vi "Native POST Multipart File Upload Example.vi"() -> ()   [LabVIEW 2017]
uses:
  <vilib>/httpClient/MultipartData.ctl
  <vilib>/httpClient/LabVIEWHTTPClient.lvlib
panel:
  out "body":string
  out "headers":string
  in  "Authentication":cluster{"Username":string, "Password":string}
  out "error out":errorcluster
  in  "FIlepath":path=path "D:/upwork/Labview-REST-API/labview-source/payload.png"
  in  "API Endpoint Url":string="https://luferau.free.beeceptor.com/upload"
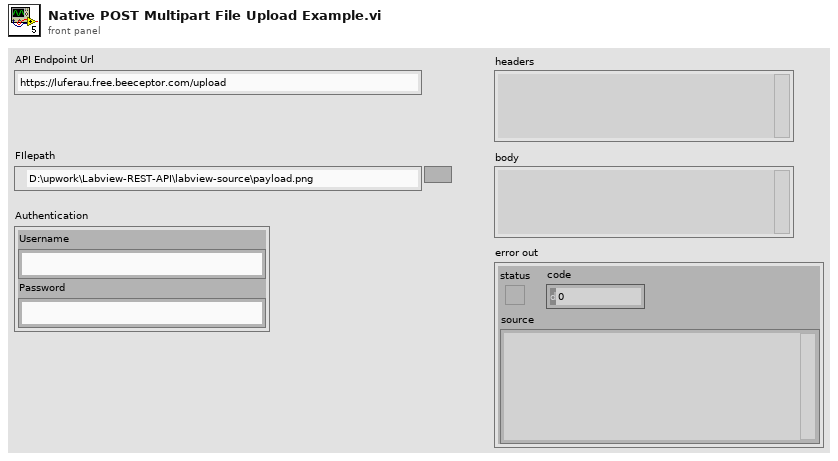
[diagram p1: front panel]
types:
  T1 = typedef "LabVIEWHTTPClient.lvlib/MultipartData.ctl" = cluster{"Name":string, "Value":string, "File":path, "Filename":string, "MIME type":string}
  T2 = typedef "LabVIEWHTTPClient.lvlib/ClientHandle.ctl" = refnum<k1>
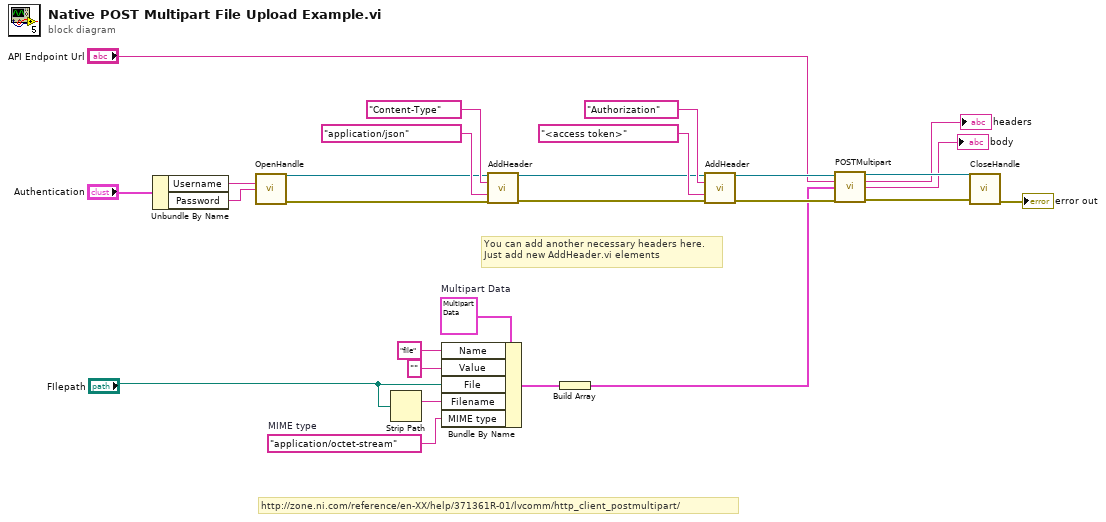
[diagram p0: block diagram]
diagram:
  w4 = "application/octet-stream"  # MIME type
  w8 = T1 {"Name"="", "Value"="", "File"=path "", "Filename"="", "MIME type"="application/octet-stream"}  # Multipart Data
  # "http://zone.ni.com/reference/en-XX/help/371361R-01/lvcomm/http_client_postmultipart/"
  # "You can add another necessary headers here.\nJust add new AddHeader.vi elements"
  n1 = Unbundle By Name("Authentication") -> ("Username"=w26:string, "Password"=w25:string)
  n2 = call <vilib>:"OpenHandle.vi"("username"=w26, "password"=w25) -> ("client handle out"=w10:T2, "error out"=w13:errorcluster)  [unwired: 12 in]
  n3 = Strip Path(path="FIlepath") -> (name=w5:string)  [unwired: 1 out]
  n4 = Bundle By Name(cluster=w8, "Name"="file", "Value"="", "File"="FIlepath", "Filename"=w5, "MIME type"=w4) -> (w3:T1)
  n5 = call <vilib>:"AddHeader.vi"("client handle"=w10, "header"="Content-Type", "value"="application/json", "error in (no error)"=w13) -> ("client handle out"=w11:T2, "error out"=w12:errorcluster)  [unwired: 10 in]
  n6 = Build Array(w3) -> (w1:T1[])
  n7 = call <vilib>:"AddHeader.vi"("client handle"=w11, "header"="Authorization", "value"="<access token>", "error in (no error)"=w12) -> ("client handle out"=w21:T2, "error out"=w20:errorcluster)  [unwired: 10 in]
  n8 = call <vilib>:"POSTMultipart.vi"("client handle"=w21, "url"="API Endpoint Url", "data"=w1, "error in (no error)"=w20) -> ("client handle out"=w19:T2, "headers"=→"headers":string, "body"=→"body":string, "error out"=w18:errorcluster)  [unwired: 8 in]
  n9 = call <vilib>:"CloseHandle.vi"("client handle"=w19, "error in (no error)"=w18) -> ("error out"=→"error out":errorcluster)  [unwired: 13 in]
